vi "CLD 7 Time Stamp to String Challenge Solution.vi"(8 "Error In":errorcluster) -> (0 "Error Out":errorcluster, 3 "Code String Out":string)   [LabVIEW 2019]
doc: "CLD 7: This exercise uses the Format Into String function."
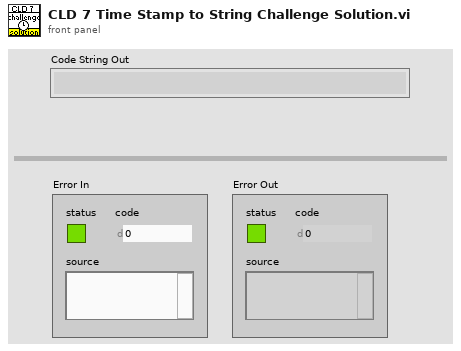
[diagram p1: front panel]
types:
  T1 = typedef "LVDateTimeRec.ctl" = cluster{"fractional second":dbl, "second":i32, "minute":i32, "hour":i32, "day of month":i32, "month":i32, "year":i32, "day of week":i32, "day of year":i32, "DST":i32}
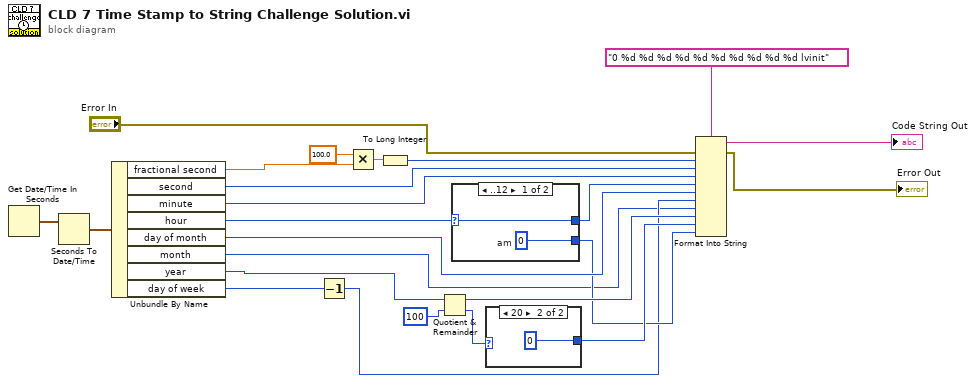
[diagram p0: block diagram]
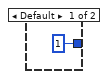
[diagram p2: hidden frame]
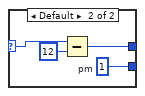
[diagram p3: hidden frame]
diagram:
  n1 = Get Date/Time In Seconds() -> (seconds since 1Jan1904=w4:timestamp)
  n2 = Seconds To Date/Time(time stamp (now)=w4) -> (date time rec=w23:T1)  [unwired: 1 in]
  n3 = Unbundle By Name(w23) -> ("fractional second"=w22:dbl, "second"=w18:i32, "minute"=w1:i32, "hour"=w17:i32, "day of month"=w15:i32, "month"=w6:i32, "year"=w14:i32, "day of week"=w8:i32)
  n4 = Decrement(x=w8) -> (x-1=w7:i32)
  n5 = Multiply(x=100.0, y=w22) -> (x*y=w20:dbl)
  n6 = To Long Integer(number=w20) -> (32bit integer=w19:i32)
  n7 = Quotient & Remainder(x=w14, y=100) -> (x-y*floor(x/y)=w12:i32, floor(x/y)=w11:i32)
  n8 = case shown="..12" w17 {
    selector: w17 -> [w26 w30]
    tunnel: [w26 w28] -> w16
    tunnel: [w25 w29] -> w9
    frame ..12 {
      w25 = 0  # am
    }
    frame Default {
      w29 = 1  # pm
      n9 = Subtract(x=w30, y=12) -> (x-y=w28:i32)
    }
  }
  n10 = case shown="20" w11 {
    tunnel: [1 ("y") 0 ("y")] -> w10
    frame Default {
    }
    frame 20 {
    }
  }
  n11 = Format Into String "Format Into String"(format string="0 %d %d %d %d %d %d %d %d %d %d lvinit", error in="Error In", w19, w18, w1, w16, w15, w7, w6, w12, w10, w9) -> (resulting string=→"Code String Out":string, error out=→"Error Out":errorcluster)  [unwired: 1 in]
